vi "ReadVIRefnum.vi"(8 "error in (no error)":errorcluster, 11 "Blacklist in":refnum<class "Blacklist.lvclass">) -> (0 "error out":errorcluster, 2 "VI Refnum":refnum<vi>, 3 "Blacklist out":refnum<class "Blacklist.lvclass">)   [LabVIEW 2014, in "lvbuildsecurity.lvlib" / "Blacklist.lvclass"]
uses:
  Blacklist.lvclass
  Blacklist.lvclass/Blacklist.ctl
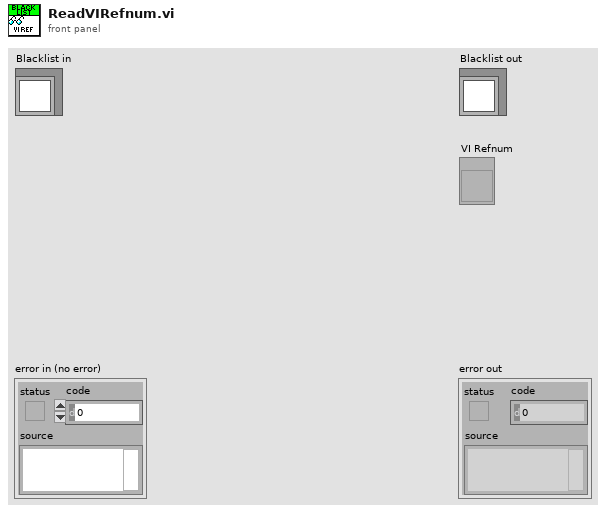
[diagram p1: front panel]
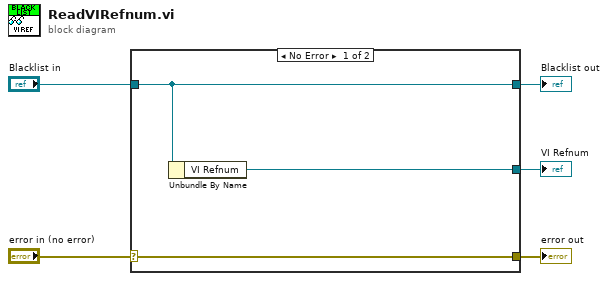
[diagram p0: block diagram]
diagram:
  n1 = case shown="No Error" "error in (no error)" {
    selector: "error in (no error)" -> [w8 w9]
    tunnel: [w8 w9] -> w4
    tunnel: [w7 w10] -> w2
    tunnel: "Blacklist in" -> [w7 w10]
    tunnel: [w6 _] -> w1
    frame No Error {
      n2 = Unbundle By Name(w7) -> ("VI Refnum"=w6:refnum<vi>)
    }
    frame Error {
    }
  }
  "error out" <- w4
  "Blacklist out" <- w2
  "VI Refnum" <- w1
